vi "String - Boolean Ref Color.vi"(5 "Bool Refnum":refnum<vi>) -> (2 "Color (U32 String)":string)   [LabVIEW 2013]
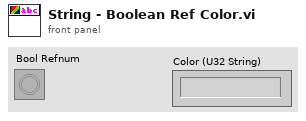
[diagram p1: front panel]
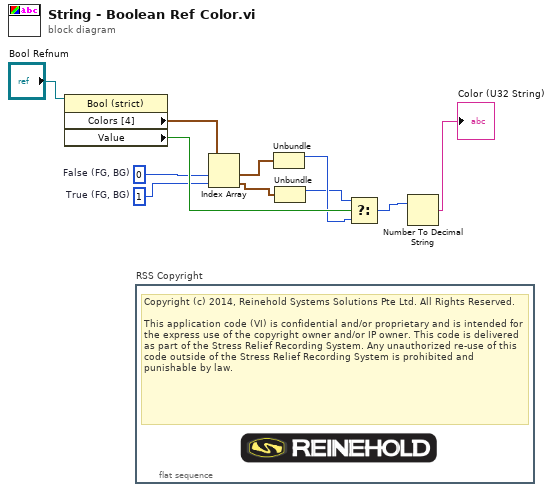
[diagram p0: block diagram]
diagram:
  w1 = 1  # True (FG, BG)
  w2 = 0  # False (FG, BG)
  n1 = property class="Bool (strict)"(reference="Bool Refnum") -> ("Colors [4]"=w8:cluster{u32, u32}[], "Value"=w6:bool)  [unwired: 1 in, 2 out]
  n2 = flat-sequence "RSS Copyright" {
    frame #0 {
      # "Copyright (c) 2014, Reinehold Systems Solutions Pte Ltd. All Rights Reserved.\n\nThis application code (VI) is confidential and/or proprietary and is intended for the express use of the copyright owner and/or IP owner. This code is delivered as part of the Stress Relief Recording System. Any unauthorized re-use of this code outside of the Stress Relief Recording System is prohibited and punishable by law."
    }
  }
  n3 = Index Array(array=w8, index #1=w2, index #2=w1) -> (element #1=w10:cluster{u32, u32}, element #2=w4:cluster{u32, u32})
  n4 = Unbundle(w10) -> (w5:u32)  [unwired: 1 out]
  n5 = Unbundle(w4) -> (w3:u32)  [unwired: 1 out]
  n6 = Select(t=w3, s=w6, f=w5) -> (s? t:f=w7:u32)
  n7 = Number To Decimal String(number=w7) -> (decimal integer string=→"Color (U32 String)":string)  [unwired: 1 in]
